vi "Teleop.vi"(10 "Match Info":T1={"Autonomous Elapsed Seconds"=0.0, "TeleOp Elapsed Seconds"=0.0, "Disabled Elapsed Seconds"=0.0, "Visited Autonomous"=FALSE, "Visited TeleOp"=FALSE, "Visited Disabled"=FALSE, "Autonomous Settings"={"Autonomous Style"=enum."Independent", "VI Refnum"=refnum}}, 11 "Call Context":T2) -> ()   [LabVIEW 2015]
doc: "This VI is called for each TeleOp packet received from the DS where the robot is not disabled. It is often used to read from the joysticks and update I/O or to update setpoints for timed control loops. It should complete and return within 20 milliseconds or it may miss DS packets."
uses:
  <vilib>/Rock Robotics/WPI/DriverStation/WPI_DriverStationDerivedRobotMode.ctl
  <vilib>/Rock Robotics/WPI/DriverStation/WPI_DriverStationMatch Info.ctl
  <vilib>/Rock Robotics/WPI/Utilities/WPI_GetSetVariantRefNum.vi
  <vilib>/Rock Robotics/Network Tables/NT Write Boolean Array.vi
  <vilib>/Rock Robotics/Network Tables/NT Write Numeric Array.vi
  <vilib>/Rock Robotics/Network Tables/NT Write Boolean.vi
  Robot Global Data.vi
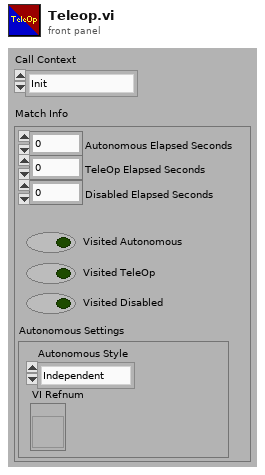
[diagram p1: front panel]
types:
  T1 = typedef "WPI_DriverStationMatch Info.ctl" = cluster{"Autonomous Elapsed Seconds":dbl, "TeleOp Elapsed Seconds":dbl, "Disabled Elapsed Seconds":dbl, "Visited Autonomous":bool, "Visited TeleOp":bool, "Visited Disabled":bool, "Autonomous Settings":cluster{"Autonomous Style":enum16{"Iterative", "Independent"}, "VI Refnum":refnum<vi>}}
  T2 = typedef "WPI_DriverStationDerivedRobotMode.ctl" = enum16{"Init", "Execute", "Stop"}
  T3 = enum16{"Start", "Start Shooter Wheels", "Fire", "Stop Shooter Wheels"}
  T4 = typedef "WPI_JoystickDevRef.ctl" = cluster{"Device":T5}
  T5 = typedef "WPI_JoystickDeviceEnum.ctl" = enum16{"USB 0", "USB 1", "USB 2", "USB 3", "USB 4", "USB 5"}
  T6 = typedef "WPI_PotentiometerDevRef.ctl" = cluster{"DevStatus":errorcluster, "Analog Channel":T7, "Invert Output":bool}
  T7 = typedef "FPGA_AIChannel.ctl" = enum8{"AI 0", "AI 1", "AI 2", "AI 3", "AI MXP 0", "AI MXP 1", "AI MXP 2", "AI MXP 3", "Invalid"}
  T8 = cluster{"Axes[0]":dbl, "Axes[1]":dbl, "Axes[2]":dbl, "Axes[3]":dbl, "Axes[4]":dbl, "Axes[5]":dbl, "Axes[6]":dbl, "Axes[7]":dbl, "Axes[8]":dbl}
  T9 = cluster{"Buttons[0]":bool, "Buttons[1]":bool, "Buttons[2]":bool, "Buttons[3]":bool, "Buttons[4]":bool, "Buttons[5]":bool, "Buttons[6]":bool, "Buttons[7]":bool, "Buttons[8]":bool}
  T10 = cluster{"POVs[0]":i16, "POVs[1]":i16, "POVs[2]":i16, "POVs[3]":i16, "POVs[4]":i16, "POVs[5]":i16, "POVs[6]":i16, "POVs[7]":i16, "POVs[8]":i16}
  T11 = typedef "WPI_MotorControlDeviceRef.ctl" = cluster{"DeviceStatus":errorcluster, "Type":T12, "PWM":cluster{"PWM Channel":T13, "DeadBand":T14}, "CAN":cluster{"Device Number":u8, "Control Mode":T15, "Semaphore":T16, "Max Vout":dbl, "TalonSRX Control Mode":T17}, "Invert":bool}
  T12 = typedef "WPI_MotorControlType.ctl" = enum16{"PWM", "CAN", "CANTalonSRX"}
  T13 = typedef "FPGA_DIOPWMChannel.ctl" = enum8{"PWM 0", "PWM 1", "PWM 2", "PWM 3", "PWM 4", "PWM 5", "PWM 6", "PWM 7", "PWM 8", "PWM 9", "PWM MXP 0", "PWM MXP 1", "PWM MXP 2", "PWM MXP 3", "PWM MXP 4", "PWM MXP 5", "PWM MXP 6", "PWM MXP 7", "PWM MXP 8", "PWM MXP 9", "Invalid"}
  T14 = typedef "WPI_PWMDeadband.ctl" = cluster{"Name":string, "maxPositivePwm":i32, "minPositivePwm":i32, "centerPwm":i32, "maxNegativePwm":i32, "minNegativePwm":i32, "angularRange":u16}
  T15 = typedef "WPI_CANJaguar_ControlMode.ctl" = enum8{"Percent VBus", "Current", "Speed", "Position", "Voltage"}
  T16 = typedef "Semaphore RefNum" = refnum<k1>
  T17 = typedef "WPI_CANTalonSRX_APIControlMode.ctl" = enum8{"Percent VBus", "Speed", "Position", "Slave", "Unchanged / Invalid", "Voltage Compensation", "Current", "Motion Profile"}
  T18 = typedef "WPI_SwitchDevRef.ctl" = cluster{"DevStatus":errorcluster, "DIO Channel":T19, "CntIndex":T20, "Normally Closed":bool}
  T19 = typedef "FPGA_DIOChannel.ctl" = enum8{"DIO 0", "DIO 1", "DIO 2", "DIO 3", "DIO 4", "DIO 5", "DIO 6", "DIO 7", "DIO 8", "DIO 9", "DIO MXP 0", "DIO MXP 1", "DIO MXP 2", "DIO MXP 3", "DIO MXP 4", "DIO MXP 5", "DIO MXP 6", "DIO MXP 7", "DIO MXP 8", "DIO MXP 9", "DIO MXP 10", "DIO MXP 11", "DIO MXP 12", "DIO MXP 13", "DIO MXP 14", "DIO MXP 15", "Invalid"}
  T20 = typedef "FPGA_CounterCtrSystemIndex.ctl" = enum8{"Ctr 0", "Ctr 1", "Ctr 2", "Ctr 3", "Ctr 4", "Ctr 5", "Ctr 6", "Ctr 7", "Invalid"}
  T21 = typedef "WPI_RobotDriveDevRef.ctl" = cluster{"DevStatus":errorcluster, "Motors[]":T11[], "Square Inputs":bool, "Max Output":dbl}
  T22 = typedef "WPI_ServoDeviceRef.ctl" = cluster{"DeviceStatus":errorcluster, "PWM Channel":T13, "DeadBand":T14}
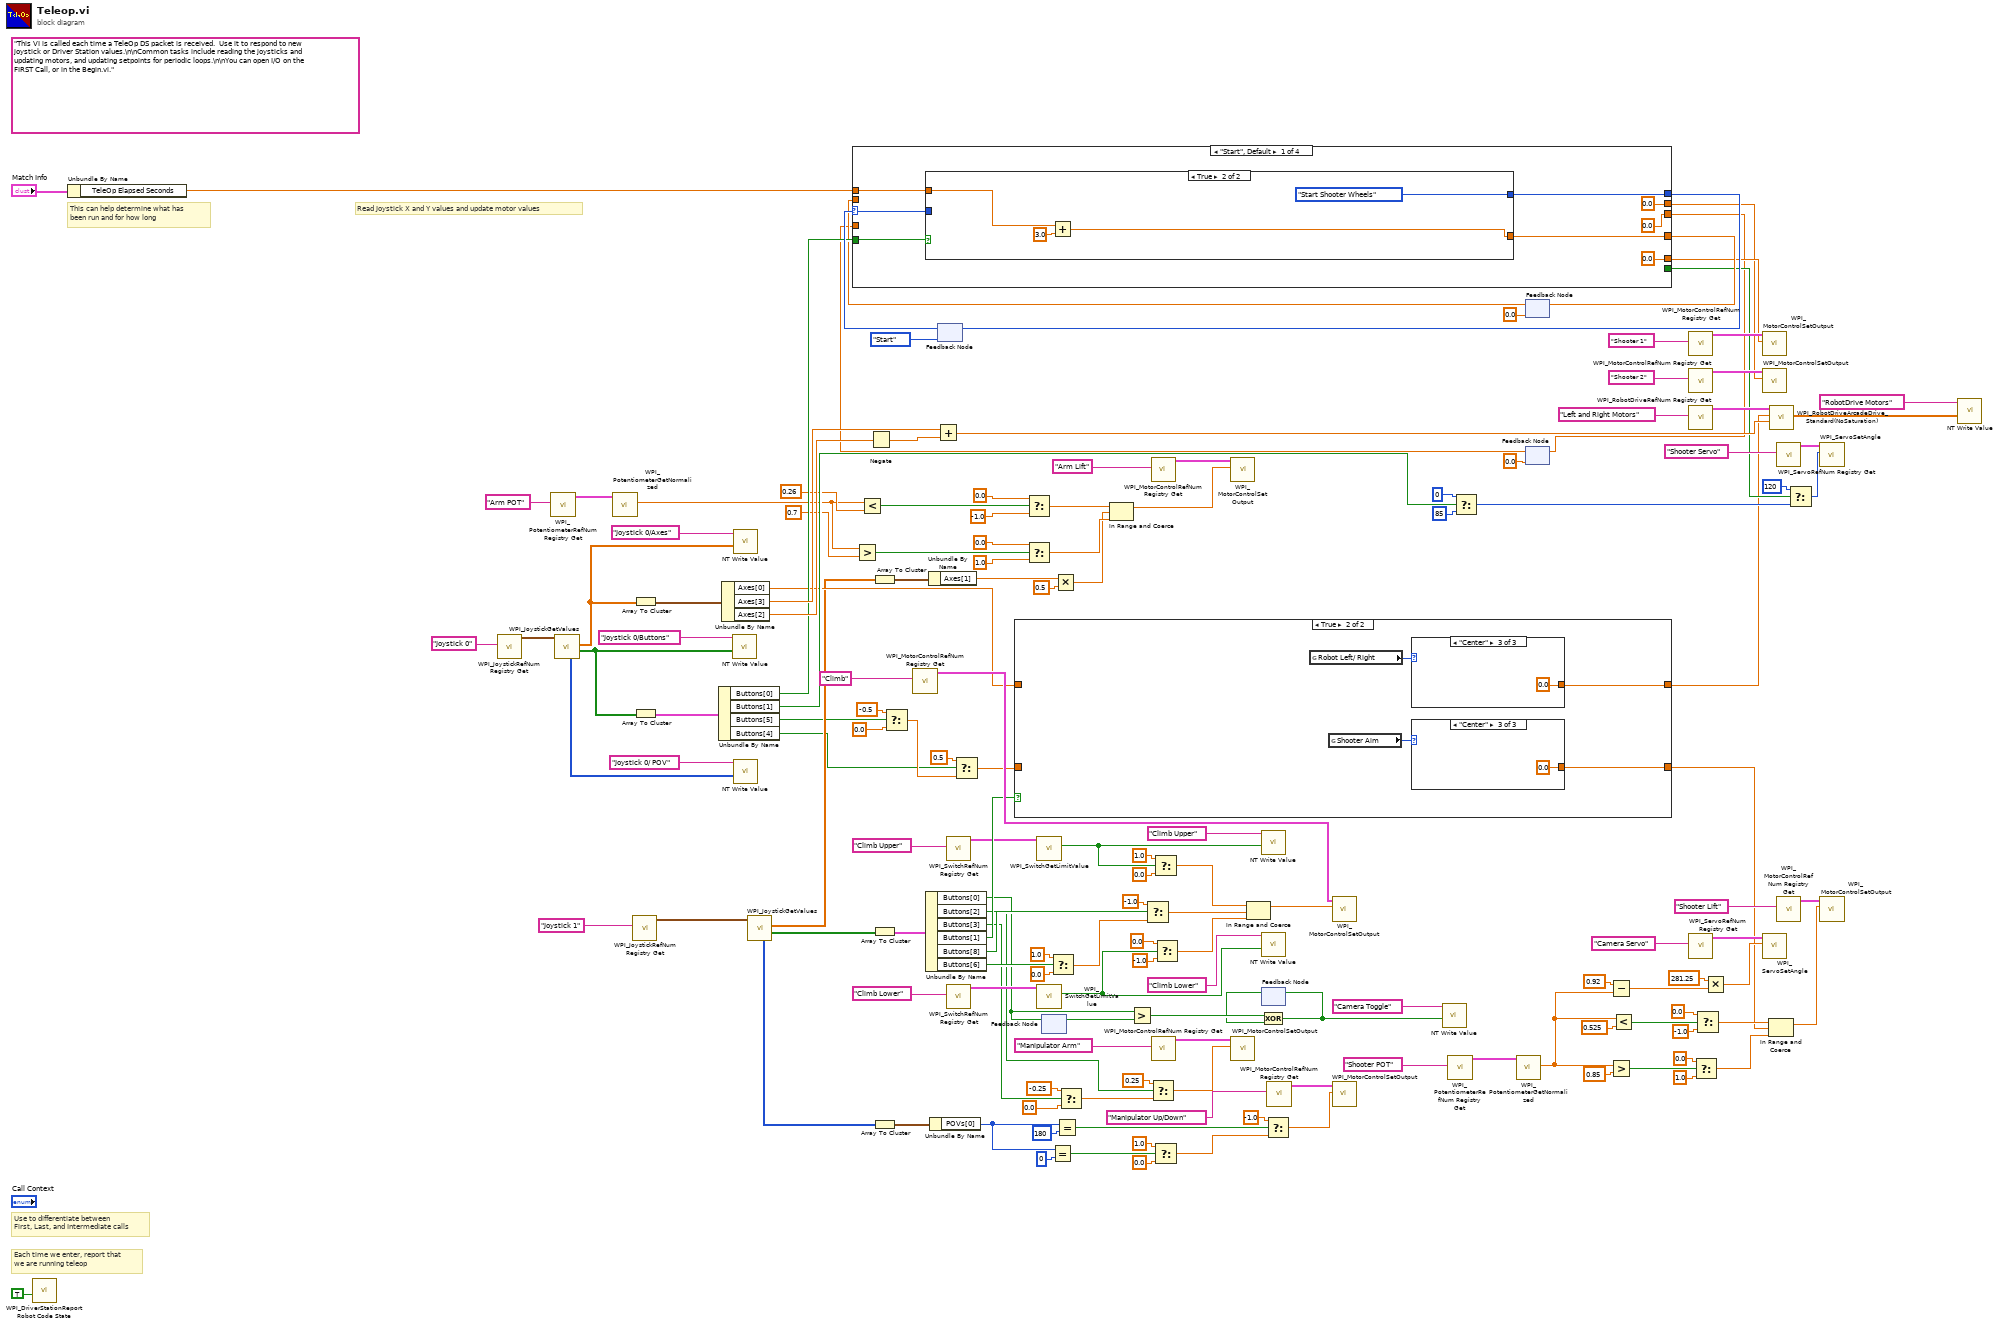
[diagram p0: block diagram]
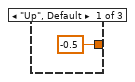
[diagram p3: hidden frame]
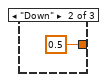
[diagram p4: hidden frame]
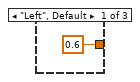
[diagram p5: hidden frame]
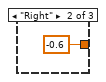
[diagram p6: hidden frame]
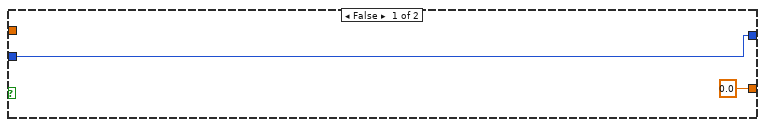
[diagram p7: hidden frame]
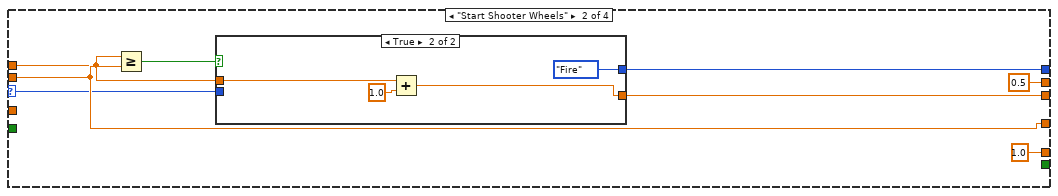
[diagram p8: hidden frame]
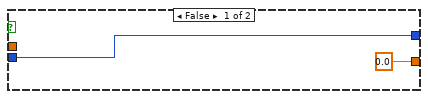
[diagram p9: hidden frame]
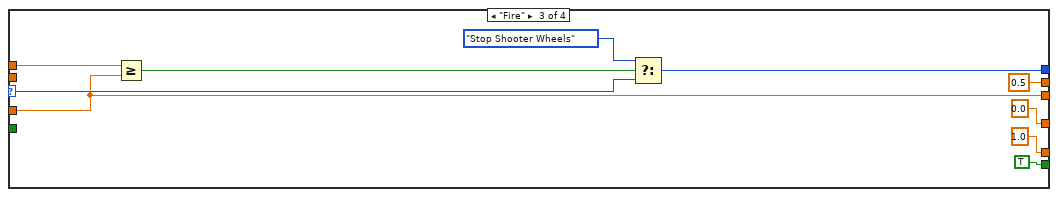
[diagram p10: hidden frame]
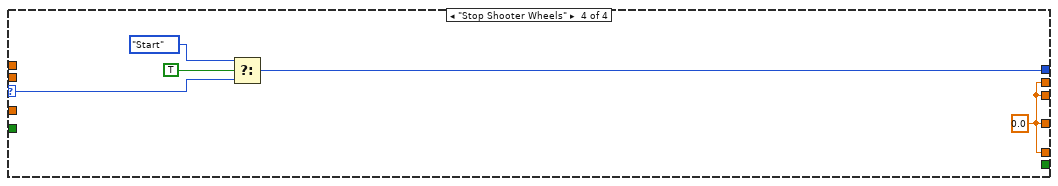
[diagram p11: hidden frame]
diagram:
  (unwired) "This VI is called each time a TeleOp DS packet is received.  Use it to respond to new joystick or Driver Station values.\n\nCommon tasks include reading the joysticks and updating motors, and updating setpoints for periodic loops.\n\nYou can open I/O on the FIRST Call, or in the Begin.vi."
  # "Each time we enter, report that\nwe are running teleop"
  # "Use to differentiate between\nFirst, Last, and Intermediate calls"
  # "This can help determine what has\nbeen run and for how long"
  # "Read Joystick X and Y values and update motor values"
  n1 = call <vilib>:"WPI_DriverStationReport Robot Code State.vi"("TeleOp"=TRUE ("Autonomous")) -> ()  [unwired: 10 in, 1 out]
  n2 = Unbundle By Name("Match Info") -> ("TeleOp Elapsed Seconds"=w129:dbl)
  n3 = call <vilib>:"WPI_JoystickRefNum Registry Get.vi"("refnum name"="Joystick 0") -> ("JoystickDevRef"=w153:T4)  [unwired: 1 in, 9 out]
  n4 = call <vilib>:"WPI_PotentiometerRefNum Registry Get.vi"("refnum name"="Arm POT") -> ("PotDevRef"=w45:T6)  [unwired: 9 in, 1 out]
  n5 = call <vilib>:"WPI_JoystickGetValues.vi"("JoystickDevRef"=w153) -> ("Buttons"=w130:bool[], "Axes"=w147:dbl[], "POVs"=w26:i16[])  [unwired: 6 in, 2 out]
  n6 = call <vilib>:"WPI_PotentiometerGetNormalized.vi"("PotDevRef"=w45) -> ("Normalized Value"=w47:dbl)  [unwired: 8 in, 2 out]
  n7 = call <vilib>:"WPI_JoystickRefNum Registry Get.vi"("refnum name"="Joystick 1") -> ("JoystickDevRef"=w110:T4)  [unwired: 9 in, 1 out]
  n8 = Array To Cluster(array=w147) -> (cluster=w146:T8)
  n9 = Array To Cluster(array=w130) -> (cluster=w131:T9)
  n10 = Unbundle By Name(w131) -> ("Buttons[0]"=w127:bool, "Buttons[1]"=w116:bool, "Buttons[5]"=w23:bool, "Buttons[4]"=w22:bool)
  n11 = Unbundle By Name(w146) -> ("Axes[0]"=w104:dbl, "Axes[3]"=w143:dbl, "Axes[2]"=w145:dbl)
  n12 = call-poly <vilib>:"NT Write Value.vi"("Boolean Array"=w130, "Name"="Joystick 0/Buttons") -> ()  [unwired: 9 in, 1 out]
  n13 = call-poly <vilib>:"NT Write Value.vi"("Numeric Array"=w147, "Name"="Joystick 0/Axes") -> ()  [unwired: 9 in, 1 out]
  n14 = call-poly <vilib>:"NT Write Value.vi"("Numeric Array"=w26, "Name"="Joystick 0/ POV") -> ()  [unwired: 9 in, 1 out]
  n15 = call <vilib>:"WPI_JoystickGetValues.vi"("JoystickDevRef"=w110) -> ("Buttons"=w101:bool[], "Axes"=w102:dbl[], "POVs"=w33:i16[])  [unwired: 6 in, 2 out]
  n16 = Greater?(x=w47, y=0.7) -> (0:w35:bool)
  n17 = Less?(x=w47, y=0.26) -> (x < y?=w36:bool)
  n18 = Negate(x=w145) -> (-x=w144:dbl)
  n19 = Array To Cluster(array=w102) -> (cluster=w100:T8)
  n20 = Array To Cluster(array=w101) -> (cluster=w99:T9)
  n21 = Array To Cluster(array=w33) -> (cluster=w32:T10)
  n22 = Select(t=-0.5, s=w23, f=0.0) -> (s? t:f=w24:dbl)
  n23 = call <vilib>:"WPI_MotorControlRefNum Registry Get.vi"("refnum name"="Climb") -> ("MotorControlDevRef"=w105:T11)  [unwired: 9 in, 1 out]
  n24 = Unbundle By Name(w99) -> ("Buttons[0]"=w10:bool, "Buttons[2]"=w29:bool, "Buttons[3]"=w30:bool, "Buttons[1]"=w98:bool, "Buttons[8]"=w96:bool, "Buttons[6]"=w95:bool)
  n25 = Unbundle By Name(w100) -> ("Axes[1]"=w107:dbl)
  n26 = Unbundle By Name(w32) -> ("POVs[0]"=w16:i16)
  n27 = Add(x=w143, y=w144) -> (x+y=w142:dbl)
  n28 = feedback #1(T3."Start") -> (w133:T3)
  n29 = call <vilib>:"WPI_SwitchRefNum Registry Get.vi"("refnum name"="Climb Upper") -> ("SwitchDevRef"=w77:T18)  [unwired: 9 in, 1 out]
  n30 = call <vilib>:"WPI_SwitchRefNum Registry Get.vi"("refnum name"="Climb Lower") -> ("SwitchDevRef"=w76:T18)  [unwired: 9 in, 1 out]
  n31 = Select(t=0.5, s=w22, f=w24) -> (s? t:f=w2:dbl)
  n32 = case shown="True" w98 {
    tunnel: w104 -> [w159 _]
    tunnel: [w159 w162] -> w103
    tunnel: w2 -> [w158 _]
    tunnel: [w158 w160] -> w1
    frame False {
    }
    frame True {
      n33 = global read "Robot Global Data.vi" "Robot Left/ Right"() -> (w163:enum16{"Left", "Right", "Center"})
      n34 = global read "Robot Global Data.vi" "Shooter Aim"() -> (w161:enum16{"Up", "Down", "Center"})
      n35 = case shown="\"Center\"" w163 {
        tunnel: [0.6 -0.6 0.0] -> w162
        frame "Left", Default {
        }
        frame "Right" {
        }
        frame "Center" {
        }
      }
      n36 = case shown="\"Center\"" w161 {
        tunnel: [-0.5 0.5 0.0] -> w160
        frame "Up", Default {
        }
        frame "Down" {
        }
        frame "Center" {
        }
      }
    }
  }
  n37 = Select(t=0.0, s=w36, f=-1.0) -> (s? t:f=w40:dbl)
  n38 = Select(t=0.0, s=w35, f=1.0) -> (s? t:f=w41:dbl)
  n39 = call <vilib>:"WPI_SwitchGetLimitValue.vi"("SwitchDevRef"=w77) -> ("Switch Pressed"=w74:bool)  [unwired: 8 in, 2 out]
  n40 = call <vilib>:"WPI_SwitchGetLimitValue.vi"("SwitchDevRef"=w76) -> ("Switch Pressed"=w71:bool)  [unwired: 8 in, 2 out]
  n41 = feedback #2() -> (w11:bool)  [unwired: 1 in]
  n42 = feedback-in #2(w10) -> ()
  n43 = Equal?(x=w16, y=0) -> (x = y?=w17:bool)
  n44 = Select(t=1.0, s=w95, f=0.0) -> (s? t:f=w97:dbl)
  n45 = Multiply(x=w107, y=0.5) -> (x*y=w38:dbl)
  n46 = Equal?(x=w16, y=i16 180) -> (x = y?=w18:bool)
  n47 = Select(t=-0.25, s=w30, f=0.0) -> (s? t:f=w63:dbl)
  n48 = In Range and Coerce(upper limit=w40, x=w38, lower limit=w41) -> (coerced(x)=w37:dbl)  [unwired: 1 out]
  n49 = Greater?(x=w10, y=w11) -> (0:w14:bool)
  n50 = Select(t=-1.0, s=w96, f=w97) -> (s? t:f=w84:dbl)
  n51 = call <vilib>:"WPI_MotorControlRefNum Registry Get.vi"("refnum name"="Arm Lift") -> ("MotorControlDevRef"=w108:T11)  [unwired: 9 in, 1 out]
  n52 = call <vilib>:"WPI_MotorControlRefNum Registry Get.vi"("refnum name"="Manipulator Arm") -> ("MotorControlDevRef"=w67:T11)  [unwired: 9 in, 1 out]
  n53 = Select(t=0.25, s=w29, f=w63) -> (s? t:f=w62:dbl)
  n54 = Select(t=1.0, s=w74, f=0.0) -> (s? t:f=w82:dbl)
  n55 = Select(t=1.0, s=w17, f=0.0) -> (s? t:f=w86:dbl)
  n56 = Select(t=0.0, s=w71, f=-1.0) -> (s? t:f=w81:dbl)
  n57 = call <vilib>:"WPI_MotorControlSetOutput.vi"("Output"=w37, "MotorControlDevRef"=w108) -> ()  [unwired: 7 in, 3 out]
  n58 = call <vilib>:"WPI_MotorControlSetOutput.vi"("Output"=w62, "MotorControlDevRef"=w67) -> ()  [unwired: 7 in, 3 out]
  n59 = In Range and Coerce(upper limit=w82, x=w84, lower limit=w81) -> (coerced(x)=w83:dbl)  [unwired: 1 out]
  n60 = call-poly <vilib>:"NT Write Value.vi"("Boolean"=w74, "Name"="Climb Upper" ("refnum name")) -> ()  [unwired: 9 in, 1 out]
  n61 = call-poly <vilib>:"NT Write Value.vi"("Boolean"=w71, "Name"="Climb Lower" ("refnum name")) -> ()  [unwired: 9 in, 1 out]
  n62 = feedback #3() -> (w12:bool)  [unwired: 1 in]
  n63 = Exclusive Or(1:w12, 2:w14) -> (0:w13:bool)
  n64 = feedback-in #3(w13) -> ()
  n65 = Select(t=-1.0, s=w18, f=w86) -> (s? t:f=w28:dbl)
  n66 = call <vilib>:"WPI_MotorControlRefNum Registry Get.vi"("refnum name"="Manipulator Up/Down") -> ("MotorControlDevRef"=w89:T11)  [unwired: 9 in, 1 out]
  n67 = call <vilib>:"WPI_MotorControlSetOutput.vi"("Output"=w83, "MotorControlDevRef"=w105) -> ()  [unwired: 7 in, 3 out]
  n68 = call <vilib>:"WPI_MotorControlSetOutput.vi"("Output"=w28, "MotorControlDevRef"=w89) -> ()  [unwired: 7 in, 3 out]
  n69 = call-poly <vilib>:"NT Write Value.vi"("Boolean"=w13, "Name"="Camera Toggle") -> ()  [unwired: 9 in, 1 out]
  n70 = call <vilib>:"WPI_PotentiometerRefNum Registry Get.vi"("refnum name"="Shooter POT") -> ("PotDevRef"=w55:T6)  [unwired: 9 in, 1 out]
  n71 = Select(t=0, s=w116, f=85) -> (s? t:f=w119:i32)
  n72 = call <vilib>:"WPI_PotentiometerGetNormalized.vi"("PotDevRef"=w55) -> ("Normalized Value"=w6:dbl)  [unwired: 8 in, 2 out]
  n73 = feedback #4(0.0) -> (w122:dbl)
  n74 = feedback #5(0.0) -> (w113:dbl)
  n75 = case shown="\"Start\", Default" w133 {
    selector: w133 -> [w177 w186 w203 w211]
    tunnel: w129 -> [w173 w185 w200 _]
    tunnel: [w176 w188 w202 w209] -> w128
    tunnel: w127 -> [w175 _ _ _]
    tunnel: [w174 w187 0.0 w212] -> w126
    tunnel: [0.0 1.0 1.0 w212] -> w124
    tunnel: [0.0 0.5 0.5 w212] -> w123
    tunnel: w122 -> [_ w187 _ _]
    tunnel: [_ _ TRUE _] -> w115
    tunnel: [0.0 w184 w198 w212] -> w114
    tunnel: w113 -> [_ _ w198 _]
    frame "Start", Default {
      n76 = case shown="True" w175 {
        tunnel: w177 -> [w179 _]
        tunnel: [w179 T3."Start Shooter Wheels"] -> w176
        tunnel: [0.0 w182] -> w174
        tunnel: w173 -> [_ w180]
        frame False {
        }
        frame True {
          n77 = Add(x=w180, y=3.0) -> (x+y=w182:dbl)
        }
      }
    }
    frame "Start Shooter Wheels" {
      n78 = Greater Or Equal?(x=w185, y=w187) -> (x >= y?=w189:bool)
      n79 = case shown="True" w189 {
        tunnel: [w193 T3."Fire"] -> w188
        tunnel: w186 -> [w193 _]
        tunnel: w185 -> [_ w196]
        tunnel: [0.0 w195] -> w184
        frame False {
        }
        frame True {
          n80 = Add(x=w196, y=1.0) -> (x+y=w195:dbl)
        }
      }
    }
    frame "Fire" {
      n81 = Greater Or Equal?(x=w200, y=w198) -> (x >= y?=w199:bool)
      n82 = Select(t=T3."Stop Shooter Wheels", s=w199, f=w203) -> (s? t:f=w202:T3)
    }
    frame "Stop Shooter Wheels" {
      w212 = 0.0
      n83 = Select(t=T3."Start", s=TRUE, f=w211) -> (s? t:f=w209:T3)
    }
  }
  n84 = feedback-in #1(w128) -> ()
  n85 = feedback-in #4(w126) -> ()
  n86 = feedback-in #5(w114) -> ()
  n87 = Subtract(x=0.92, y=w6) -> (x-y=w8:dbl)
  n88 = Greater?(x=w6, y=0.85) -> (0:w52:bool)
  n89 = Less?(x=w6, y=0.525) -> (x < y?=w53:bool)
  n90 = call <vilib>:"WPI_MotorControlRefNum Registry Get.vi"("refnum name"="Shooter 1") -> ("MotorControlDevRef"=w138:T11)  [unwired: 9 in, 1 out]
  n91 = call <vilib>:"WPI_MotorControlRefNum Registry Get.vi"("refnum name"="Shooter 2") -> ("MotorControlDevRef"=w139:T11)  [unwired: 9 in, 1 out]
  n92 = call <vilib>:"WPI_RobotDriveRefNum Registry Get.vi"("refnum name"="Left and Right Motors") -> ("RobotDriveDevRef"=w155:T21)  [unwired: 1 in, 9 out]
  n93 = call <vilib>:"WPI_ServoRefNum Registry Get.vi"("refnum name"="Camera Servo") -> ("ServoDeviceRef"=w5:T22)  [unwired: 9 in, 1 out]
  n94 = Select(t=0.0, s=w52, f=1.0) -> (s? t:f=w60:dbl)
  n95 = Select(t=0.0, s=w53, f=-1.0) -> (s? t:f=w25:dbl)
  n96 = Multiply(x=281.25, y=w8) -> (x*y=w3:dbl)
  n97 = call <vilib>:"WPI_MotorControlSetOutput.vi"("Output"=w124, "MotorControlDevRef"=w138) -> ()  [unwired: 7 in, 3 out]
  n98 = call <vilib>:"WPI_MotorControlSetOutput.vi"("Output"=w123, "MotorControlDevRef"=w139) -> ()  [unwired: 7 in, 3 out]
  n99 = call <vilib>:"WPI_ServoSetAngle.vi"("Angle"=w3, "ServoDeviceRef"=w5) -> ()  [unwired: 8 in, 2 out]
  n100 = In Range and Coerce(upper limit=w25, x=w1, lower limit=w60) -> (coerced(x)=w61:dbl)  [unwired: 1 out]
  n101 = call <vilib>:"WPI_RobotDriveArcadeDrive_Standard(NoSaturation).vi"("Y axis value"=w142, "X axis value"=w103, "RobotDriveDevRef"=w155) -> ("Motor Values"=w149:dbl[])  [unwired: 1 in, 7 out]
  n102 = call <vilib>:"WPI_ServoRefNum Registry Get.vi"("refnum name"="Shooter Servo") -> ("ServoDeviceRef"=w135:T22)  [unwired: 9 in, 1 out]
  n103 = call <vilib>:"WPI_MotorControlRefNum Registry Get.vi"("refnum name"="Shooter Lift") -> ("MotorControlDevRef"=w140:T11)  [unwired: 9 in, 1 out]
  n104 = Select(t=120, s=w115, f=w119) -> (s? t:f=w121:i32)
  n105 = call <vilib>:"WPI_ServoSetAngle.vi"("Angle"=w121, "ServoDeviceRef"=w135) -> ()  [unwired: 8 in, 2 out]
  n106 = call <vilib>:"WPI_MotorControlSetOutput.vi"("Output"=w61, "MotorControlDevRef"=w140) -> ()  [unwired: 7 in, 3 out]
  n107 = call-poly <vilib>:"NT Write Value.vi"("Numeric Array"=w149, "Name"="RobotDrive Motors") -> ()  [unwired: 9 in, 1 out]
